vi "Strip Spartan SN.vi"(1 "SN 2":string) -> (0 "SN":string)   [LabVIEW 2011]
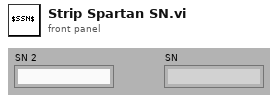
[diagram p1: front panel]
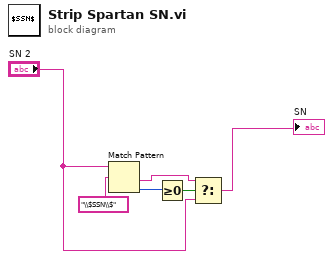
[diagram p0: block diagram]
diagram:
  n1 = Match Pattern(string="SN 2", regular expression="\\$SSN\\$") -> (after substring=w4:string, offset past match=w2:i32)  [unwired: 3 out]
  n2 = Greater Or Equal To 0?(x=w2) -> (x >= 0?=w3:bool)
  n3 = Select(t=w4, s=w3, f="SN 2") -> (s? t:f=→"SN":string)
